vi "initInputs.vi"(5 "index":i32, 6 "error in":errorcluster, 9 "Control Terminal in":refnum<class "ControlTerminal.lvclass">) -> (0 "error out":errorcluster, 3 "Control Terminal out":refnum<class "ControlTerminal.lvclass">, 4 "initValues":string)   [LabVIEW 2014, in "ControlTerminal.lvclass"]
uses:
  ControlTerminal.lvclass
  <vilib>/Utility/error.llb/whitespace.ctl
  Python/Parsing/Python Functions.lvlib
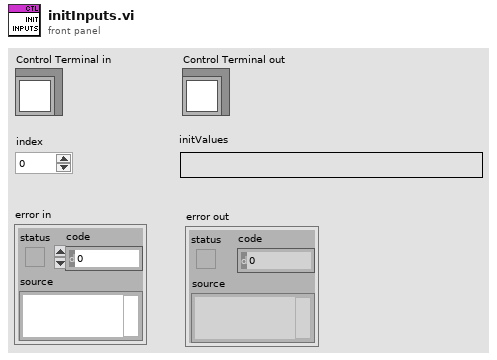
[diagram p1: front panel]
types:
  T1 = typedef "whitespace.ctl" = u16
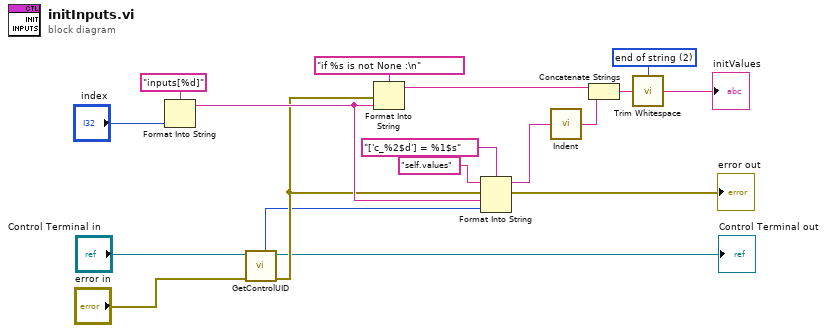
[diagram p0: block diagram]
diagram:
  w12 = T1 2 items=["both", "start of string", "end of string"] ("location (both)")
  n1 = Format Into String(format string="inputs[%d]", "index") -> (resulting string=w14:string)  [unwired: 2 in, 1 out]
  n2 = call "GetControlUID.vi"("error in"="error in", "Control Terminal in"="Control Terminal in") -> ("error out"=w5:errorcluster, "Control Terminal out"=→"Control Terminal out":refnum<class "ControlTerminal.lvclass">, "control UID"=w2:i32)  [unwired: 5 in]
  n3 = Format Into String(format string="if %s is not None :\n", error in=w5, w14) -> (resulting string=w8:string)  [unwired: 1 in, 1 out]
  n4 = Format Into String(format string="['c_%2$d'] = %1$s", initial string="self.values", error in=w5, w14, w2) -> (resulting string=w9:string, error out=→"error out":errorcluster)
  n5 = call "Indent.vi"("string in"=w9) -> ("string out"=w7:string)  [unwired: 1 in]
  n6 = Concatenate Strings(w8, w7) -> (w18:string)
  n7 = call <vilib>:"Trim Whitespace.vi"("string"=w18, "location (both)"=w12) -> ("trimmed string"=→"initValues":string)
